vi "ConfigureSubpanelPaths.vi"(8 "error in (no error)":errorcluster, 10 "Subpanel Paths":path[](array[path]), 11 "SMO.UI.MAUI in":refnum<class "SMO.UI.MAUI.lvclass">) -> (0 "error out":errorcluster, 2 "Configured Subpanel Paths":path[](array[path]), 3 "SMO.UI.MAUI out":refnum<class "SMO.UI.MAUI.lvclass">)   [LabVIEW 2020, in "SMO.UI.MAUI.lvclass"]
uses:
  SMO.UI.MAUI.lvclass
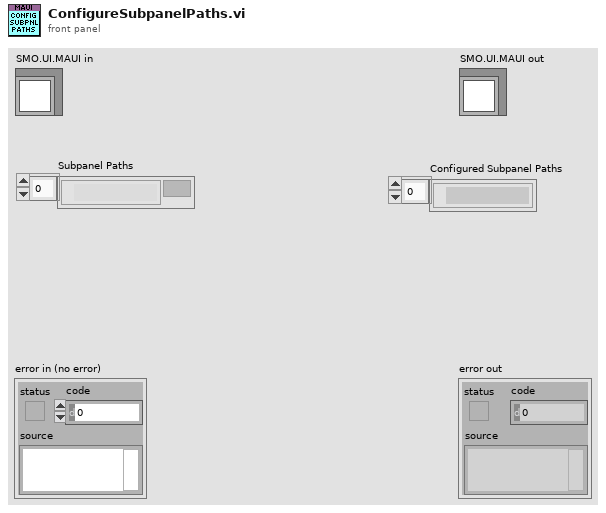
[diagram p1: front panel]
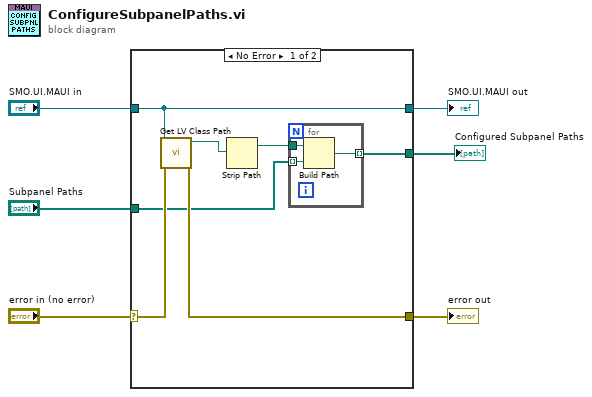
[diagram p0: block diagram]
diagram:
  n1 = case shown="No Error" "error in (no error)" {
    selector: "error in (no error)" -> [w12 w18]
    tunnel: [w11 w18] -> w5
    tunnel: [w13 w17] -> w3
    tunnel: "SMO.UI.MAUI in" -> [w13 w17]
    tunnel: "Subpanel Paths" -> [w8 _]
    tunnel: [w7 _] -> w1
    frame No Error {
      n2 = call <vilib>:"Get LV Class Path.vi"("error in (no error)"=w12, "object"=w13) -> ("error out"=w11:errorcluster, "class path"=w10:path)  [unwired: 8 in]
      n3 = Strip Path(path=w10) -> (stripped path=w9:path)  [unwired: 1 out]
      n4 = for {
        tunnel: w9 -> [w16]
        tunnel: w8 -> [w15] mode=indexing
        tunnel: [w14] -> w7 mode=indexing
        n5 = Build Path(base path=w16, name or relative path=w15) -> (appended path=w14:path)
      }
    }
    frame Error {
    }
  }
  "error out" <- w5
  "SMO.UI.MAUI out" <- w3
  "Configured Subpanel Paths" <- w1
